vi "Hardware_CommandSTR_gen.vi"(0 "Hardware Settings":T1={"Number Samples"=5000, "Time Between Points"=0.0, "Unit"="", "Gain2 (dB)"=20, "CuttOff Freq1[MHz]"=9, "CuttOff Freq2[MHz]"=1, "Frequency"=8000000.0, "Phase"=180, "Power Level"=512, "Send Pulse"=FALSE, "Reset DDS"=FALSE, "TX CTRL"=FALSE, "RX CTRL"=FALSE, "Gain1 (dB)"=15, "Set DDS"=FALSE, "Start AQS"=FALSE} {"Gain1 (dB)" min=-5 max=45 step=1; "Power Level" max=1023 step=1; "Phase" max=270 step=90; "Frequency" min=1.0 format="%^#_6e"; "CuttOff Freq2[MHz]" min=1 max=30 step=1; "CuttOff Freq1[MHz]" min=1 max=30 step=1; "Gain2 (dB)" min=-5 max=45 step=1; "Time Between Points" min=0.0 step=1.0; "Number Samples" step=1}) -> (4 "CMD STR Array":string[](array[string]))   [LabVIEW 2011]
uses:
  Controls/Hardware Control.ctl
panel:
  in  "Send All Button":bool
  in  "On/Off 2":bool
  in  "Switch Button RX":bool
  in  "On/Off":bool
  in  "Switch Button":bool
  out "Waveform Graph":i32[][](graph)
  out "XY Graph":cluster{"magnitude":dbl[], dbl[]}(graph)
  out "XY Graph 2":cluster{"magnitude":dbl[], dbl[]}(graph)
  in  "Send Botton ADC":bool
  in  "Number Samples":u16=5000 step=1
  in  "Time Between Points":dbl min=0.0 step=1.0
  in  "ms/us Time Points":bool
  out "Real Time":ext=0.73746299999999999998
  in  "Gain (dB) 2":i8=15 min=-5 max=45 step=1
  in  "Gain (dB)":i8=20 min=-5 max=45 step=1
  in  "Numeric 2":fxp<+,12,12>
  in  "Numeric":fxp<+,12,12>
  in  "Send DAC B":bool
  in  "Send DAC A":bool
  in  "CuttOff Freq [MHz]":u8=9 min=1 max=30 step=1
  in  "CuttOff Freq[MHz]":u8=1 min=1 max=30 step=1
  in  "Send PFVGA 2":bool
  in  "Send PFVGA 1":bool
  in  "Send Pulse Botton":bool
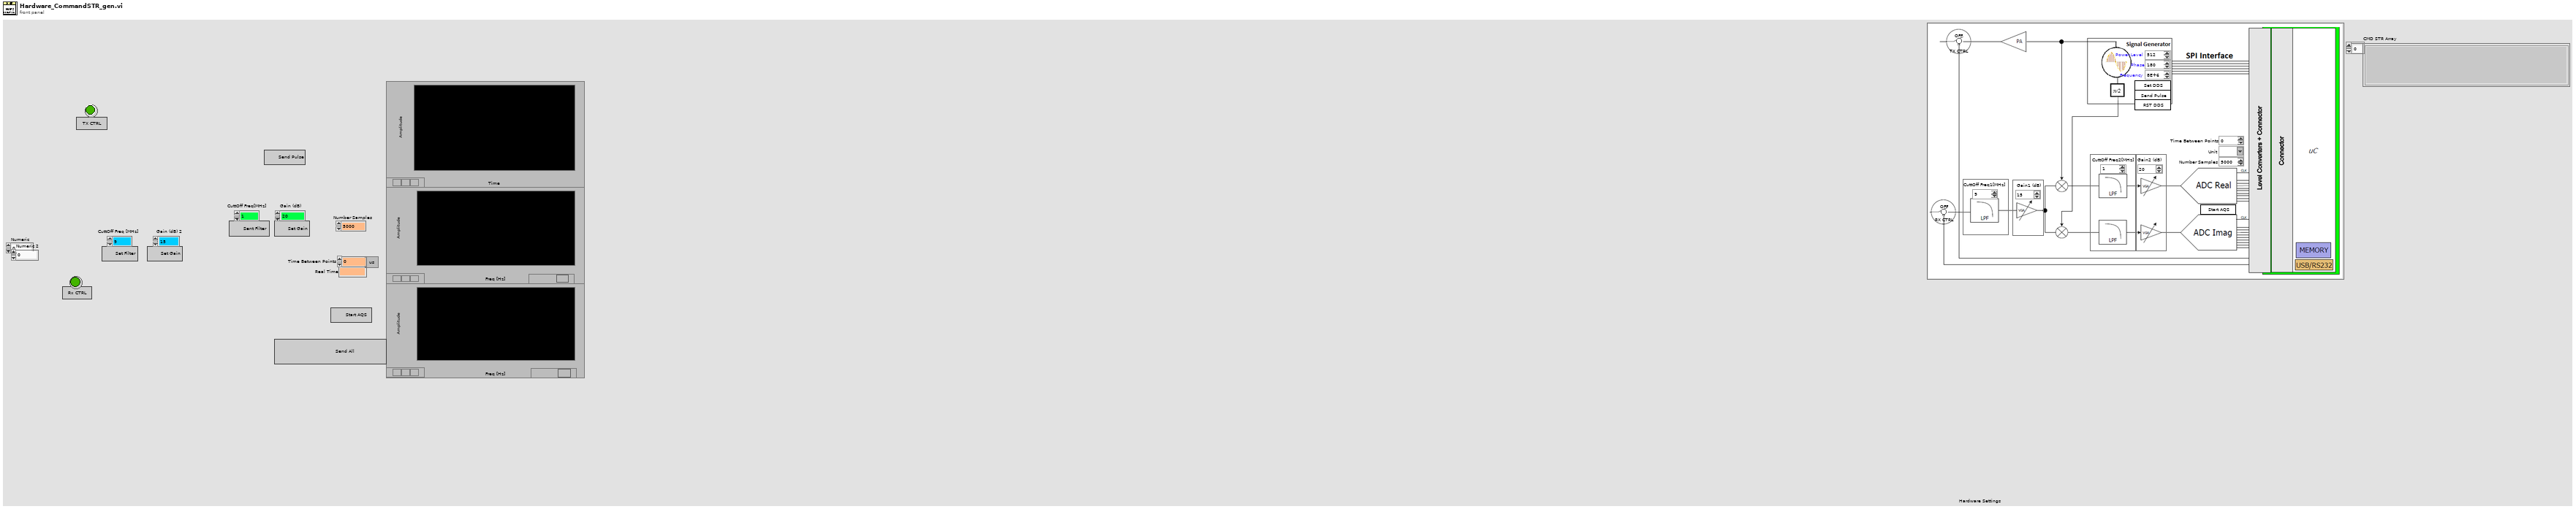
[diagram p1: front panel]
types:
  T1 = typedef "Hardware Control.ctl" = cluster{"Number Samples":u16, "Time Between Points":dbl, "Unit":string, "Gain2 (dB)":i8, "CuttOff Freq1[MHz]":u8, "CuttOff Freq2[MHz]":u8, "Frequency":dbl, "Phase":u16, "Power Level":u16, "Send Pulse":bool, "Reset DDS":bool, "TX CTRL":bool, "RX CTRL":bool, "Gain1 (dB)":i8, "Set DDS":bool, "Start AQS":bool}
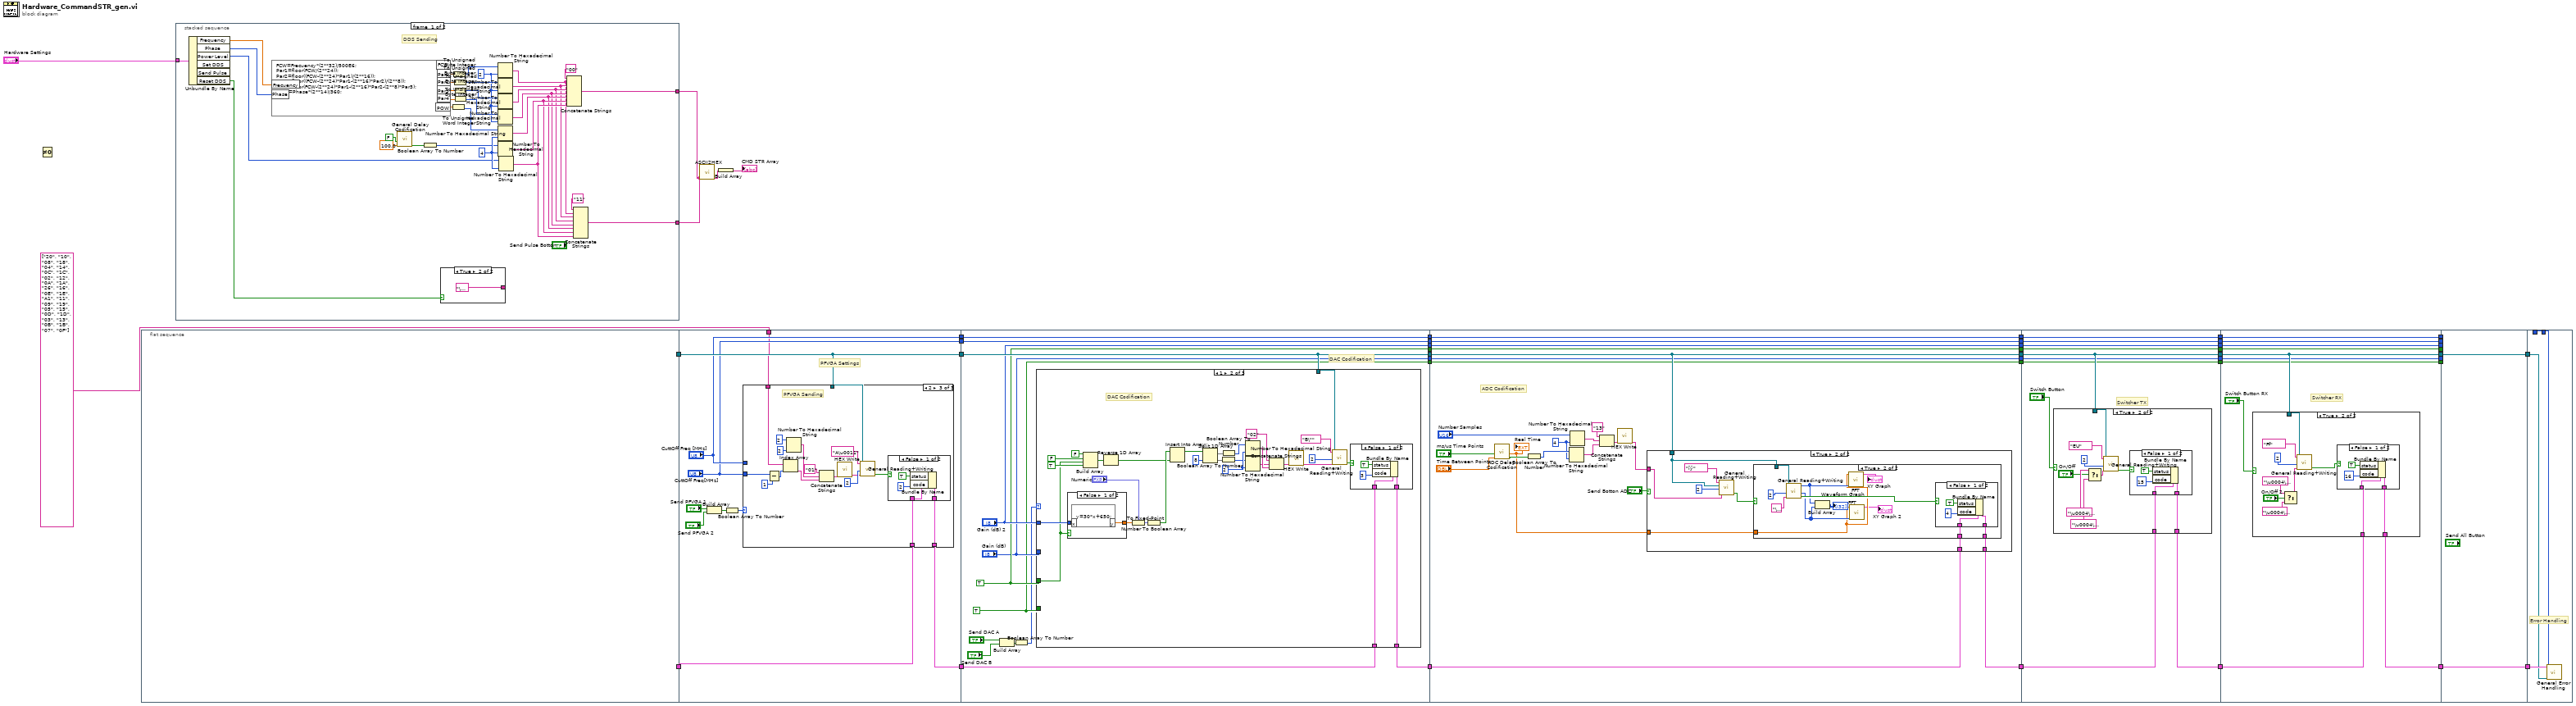
[diagram p0: block diagram]
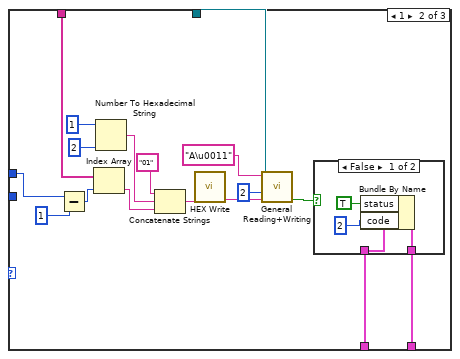
[diagram p5: hidden frame]
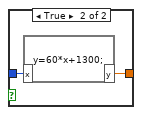
[diagram p10: hidden frame]
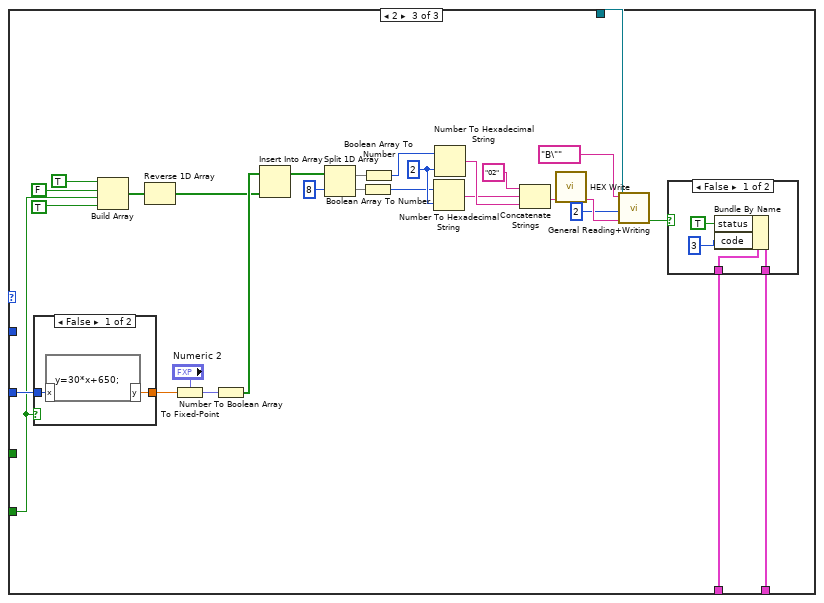
[diagram p11: hidden frame]
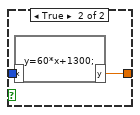
[diagram p13: hidden frame]
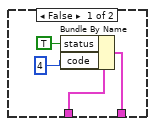
[diagram p15: hidden frame]
diagram:
  n1 = Not Equal To 0?() -> ()  [unwired: 1 in, 1 out]
  n2 = flat-sequence {
    tunnel: [_] -> w42
    tunnel: [_] -> w43
    tunnel: [w55] -> w38
    tunnel: [w54] -> w39
    tunnel: ["CuttOff Freq [MHz]"] -> w40
    tunnel: ["CuttOff Freq[MHz]"] -> w41
    tunnel: string[] ["20", "10", "08", "18", "04", "14", "0C", "1C", "02", "12", "0A", "1A", "26", "16", "0E", "1E", "A1", "11", "09", "19", "05", "15", "0D", "1D", "03", "13", "0B", "1B", "07", "0F"] ("Array") -> [w50]
    tunnel: w43 -> [w51]
    tunnel: w42 -> [w55]
    tunnel: [w113] -> w37
    tunnel: [w112] -> w36
    tunnel: [w111] -> w35
    tunnel: [w110] -> w34
    tunnel: ["Gain (dB) 2"] -> w33
    tunnel: [w108] -> w32
    tunnel: ["Gain (dB)"] -> w31
    tunnel: [w106] -> w30
    tunnel: w41 -> [w110]
    tunnel: w40 -> [w111]
    tunnel: w39 -> [w105]
    tunnel: w38 -> [w113]
    tunnel: w37 -> [w202]
    tunnel: w36 -> [w195]
    tunnel: [w205] -> w29
    tunnel: [w202] -> w28
    tunnel: w35 -> [w201]
    tunnel: [w201] -> w27
    tunnel: w34 -> [w200]
    tunnel: [w200] -> w26
    tunnel: w33 -> [w199]
    tunnel: w32 -> [w198]
    tunnel: w31 -> [w197]
    tunnel: w30 -> [w196]
    tunnel: [w199] -> w25
    tunnel: [w198] -> w24
    tunnel: [w197] -> w23
    tunnel: [w196] -> w22
    tunnel: w29 -> [w251]
    tunnel: [w250] -> w21
    tunnel: w28 -> [w249]
    tunnel: [w249] -> w20
    tunnel: w27 -> [w248]
    tunnel: w26 -> [w247]
    tunnel: [w248] -> w19
    tunnel: [w247] -> w18
    tunnel: w25 -> [w246]
    tunnel: w24 -> [w245]
    tunnel: w23 -> [w244]
    tunnel: w22 -> [w243]
    tunnel: [w246] -> w17
    tunnel: [w245] -> w16
    tunnel: [w244] -> w15
    tunnel: [w243] -> w14
    tunnel: w21 -> [w277]
    tunnel: [w276] -> w13
    tunnel: w20 -> [w275]
    tunnel: [w275] -> w12
    tunnel: w19 -> [w274]
    tunnel: w18 -> [w273]
    tunnel: [w274] -> w11
    tunnel: [w273] -> w10
    tunnel: w17 -> [w272]
    tunnel: w16 -> [w271]
    tunnel: w15 -> [w270]
    tunnel: w14 -> [w269]
    tunnel: [w272] -> w9
    tunnel: [w271] -> w8
    tunnel: [w270] -> w7
    tunnel: [w269] -> w6
    tunnel: w13 -> [w303]
    tunnel: [w303] -> w5
    tunnel: w12 -> [w295]
    tunnel: w11 -> [w302]
    tunnel: w10 -> [w301]
    tunnel: w9 -> [w300]
    tunnel: w8 -> [w299]
    tunnel: w7 -> [w298]
    tunnel: w6 -> [w297]
    tunnel: [w295] -> w4
    tunnel: w5 -> [w307]
    tunnel: w4 -> [w306]
    tunnel: _ -> [w305]
    tunnel: _ -> [w304]
    frame #0 {
    }
    frame #1 {
      # "PFVGA Settings"
      n3 = Build Array("Send PFVGA 1", "Send PFVGA 2") -> (w47:bool[])
      n4 = Boolean Array To Number(Boolean array=w47) -> (number=w46:u32)
      n5 = case shown="2" w46 {
        tunnel: w55 -> [_ w71 w92]
        tunnel: w51 -> [w56 w70 w91]
        tunnel: [w56 w69 w90] -> w54
        tunnel: "CuttOff Freq [MHz]" -> [_ w59 _]
        tunnel: w50 -> [_ w58 w82]
        tunnel: "CuttOff Freq[MHz]" -> [_ _ w81]
        frame 0, Default {
        }
        frame 1 {
          n6 = Subtract(x=w59, y=u8 1) -> (x-y=w65:u8)
          n7 = Index Array(array=w58, index=w65) -> (element=w64:string)
          n8 = Number To Hexadecimal String(1:i16 2 ("width (-)"), 2:1 ("number")) -> (0:w73:string)
          n9 = Concatenate Strings("01" ("string"), w73, w64) -> (w68:string)
          n10 = call "HEX Write.vi"("String (Normal Display)"=w68) -> ("Result string (Hex Display)"=w67:string)  [unwired: 10 in]
          n11 = call "General Reading+Writing.vi"("Write String"=w67, "Bytes to Read"=u32 2 ("Number bytes Read"), "VISA resource name"=w71, "String Seached"="A\u0011" ("search char")) -> ("Coincidence Of Character"=w60:bool)  [unwired: 4 in, 3 out]
          n12 = case shown="False" w60 {
            tunnel: w70 -> [w75 w78]
            tunnel: [w74 w78] -> w69
            frame False {
              n13 = Bundle By Name(cluster=w75, "status"=TRUE, "code"=2) -> (w74:cluster{})
            }
            frame True {
            }
          }
        }
        frame 2 {
          # "PFVGA Sending"
          n14 = Subtract(x=w81, y=u8 1) -> (x-y=w88:u8)
          n15 = Index Array(array=w82, index=w88) -> (element=w87:string)
          n16 = Number To Hexadecimal String(1:i16 2 ("width (-)"), 2:2 ("number")) -> (0:w95:string)
          n17 = Concatenate Strings("01" ("string"), w95, w87) -> (w80:string)
          n18 = call "HEX Write.vi"("String (Normal Display)"=w80) -> ("Result string (Hex Display)"=w79:string)  [unwired: 10 in]
          n19 = call "General Reading+Writing.vi"("Write String"=w79, "Bytes to Read"=u32 2 ("Number bytes Read"), "VISA resource name"=w92, "String Seached"="A\u0011" ("search char")) -> ("Coincidence Of Character"=w83:bool)  [unwired: 4 in, 3 out]
          n20 = case shown="False" w83 {
            tunnel: w91 -> [w97 w100]
            tunnel: [w96 w100] -> w90
            frame False {
              n21 = Bundle By Name(cluster=w97, "status"=TRUE, "code"=2) -> (w96:cluster{})
            }
            frame True {
            }
          }
        }
      }
    }
    frame #2 {
      w106 = TRUE ("Output Gain B")
      w108 = TRUE ("Output Gain A")
      # "DAC Codification"
      n22 = Build Array("Send DAC A", "Send DAC B") -> (w104:bool[])
      n23 = Boolean Array To Number(Boolean array=w104) -> (number=w103:u32)
      n24 = case shown="1" w103 {
        tunnel: w113 -> [_ w143 w181]
        tunnel: w105 -> [w114 w142 w180]
        tunnel: [w114 w141 w179] -> w112
        tunnel: w108 -> [_ w115 _]
        tunnel: "Gain (dB)" -> [_ _ w154]
        tunnel: "Gain (dB) 2" -> [_ w116 _]
        tunnel: w106 -> [_ _ w153]
        frame Default {
        }
        frame 1 {
          w140 = i16 2 ("width (-)")
          # "DAC Codification"
          n25 = case shown="False" w115 {
            tunnel: w116 -> [w150 w152]
            tunnel: [w149 w151] -> w129
            frame False {
              n26 = formula code="y=30*x+650;"("x"=w150) -> ("y"=w149:dbl)
            }
            frame True {
              n27 = formula code="y=60*x+1300;"("x"=w152) -> ("y"=w151:dbl)
            }
          }
          n28 = Build Array(FALSE ("element"), FALSE ("A/B"), w115, TRUE ("element")) -> (w128:bool[])
          n29 = Reverse 1D Array(array=w128) -> (reversed array=w126:bool[])
          n30 = To Fixed-Point(fixed-point type="Numeric", number=w129) -> (fixed-point=w132:fxp<+,12,12>)
          n31 = Number To Boolean Array(number=w132) -> (Boolean array=w127:bool[])
          n32 = Insert Into Array(array=w127, new element=w126) -> (w136:bool[])  [unwired: 1 in]
          n33 = Split 1D Array(array=w136, index=8) -> (first subarray=w134:bool[], second subarray=w135:bool[])
          n34 = Boolean Array To Number(Boolean array=w135) -> (number=w138:u32)
          n35 = Boolean Array To Number(Boolean array=w134) -> (number=w139:u32)
          n36 = Number To Hexadecimal String(1:w140, 2:w139) -> (0:w125:string)
          n37 = Number To Hexadecimal String(1:w140, 2:w138) -> (0:w124:string)
          n38 = Concatenate Strings("02" ("string"), w124, w125) -> (w123:string)
          n39 = call "HEX Write.vi"("String (Normal Display)"=w123) -> ("Result string (Hex Display)"=w122:string)  [unwired: 10 in]
          n40 = call "General Reading+Writing.vi"("Write String"=w122, "Bytes to Read"=u32 2 ("Number bytes Read"), "VISA resource name"=w143, "String Seached"="B\"" ("search char")) -> ("Coincidence Of Character"=w118:bool)  [unwired: 4 in, 3 out]
          n41 = case shown="False" w118 {
            tunnel: w142 -> [w145 w148]
            tunnel: [w144 w148] -> w141
            frame False {
              n42 = Bundle By Name(cluster=w145, "status"=TRUE, "code"=3) -> (w144:cluster{})
            }
            frame True {
            }
          }
        }
        frame 2 {
          w178 = i16 2 ("width (-)")
          n43 = case shown="False" w153 {
            tunnel: w154 -> [w188 w190]
            tunnel: [w187 w189] -> w167
            frame False {
              n44 = formula code="y=30*x+650;"("x"=w188) -> ("y"=w187:dbl)
            }
            frame True {
              n45 = formula code="y=60*x+1300;"("x"=w190) -> ("y"=w189:dbl)
            }
          }
          n46 = Build Array(TRUE ("element"), FALSE ("A/B"), w153, TRUE ("element")) -> (w166:bool[])
          n47 = Reverse 1D Array(array=w166) -> (reversed array=w164:bool[])
          n48 = To Fixed-Point(fixed-point type="Numeric 2", number=w167) -> (fixed-point=w170:fxp<+,12,12>)
          n49 = Number To Boolean Array(number=w170) -> (Boolean array=w165:bool[])
          n50 = Insert Into Array(array=w165, new element=w164) -> (w174:bool[])  [unwired: 1 in]
          n51 = Split 1D Array(array=w174, index=8) -> (first subarray=w172:bool[], second subarray=w173:bool[])
          n52 = Boolean Array To Number(Boolean array=w173) -> (number=w176:u32)
          n53 = Boolean Array To Number(Boolean array=w172) -> (number=w177:u32)
          n54 = Number To Hexadecimal String(1:w178, 2:w176) -> (0:w162:string)
          n55 = Number To Hexadecimal String(1:w178, 2:w177) -> (0:w163:string)
          n56 = Concatenate Strings("02" ("string"), w162, w163) -> (w161:string)
          n57 = call "HEX Write.vi"("String (Normal Display)"=w161) -> ("Result string (Hex Display)"=w160:string)  [unwired: 10 in]
          n58 = call "General Reading+Writing.vi"("Write String"=w160, "Bytes to Read"=u32 2 ("Number bytes Read"), "VISA resource name"=w181, "String Seached"="B\"" ("search char")) -> ("Coincidence Of Character"=w156:bool)  [unwired: 4 in, 3 out]
          n59 = case shown="False" w156 {
            tunnel: w180 -> [w183 w186]
            tunnel: [w182 w186] -> w179
            frame False {
              n60 = Bundle By Name(cluster=w183, "status"=TRUE, "code"=3) -> (w182:cluster{})
            }
            frame True {
            }
          }
        }
      }
    }
    frame #3 {
      w209 = i16 4 ("width (-)")
      # "ADC Codification"
      n61 = call "ADC Delay Codification.vi"("Delay"="Time Between Points", "ms/us Delay"="ms/us Time Points") -> ("Final array"=w194:bool[], "Real Time"=w191:ext)  [unwired: 8 in]
      "Real Time" <- w191
      n62 = Boolean Array To Number(Boolean array=w194) -> (number=w212:u32)
      n63 = Number To Hexadecimal String(1:w209, 2:w212) -> (0:w211:string)
      n64 = Number To Hexadecimal String(1:w209, 2:"Number Samples") -> (0:w210:string)
      n65 = Concatenate Strings("13" ("string"), w210, w211) -> (w204:string)
      n66 = call "HEX Write.vi"("String (Normal Display)"=w204) -> ("Result string (Hex Display)"=w203:string)  [unwired: 10 in]
      n67 = case shown="True" "Send Botton ADC" {
        tunnel: w203 -> [_ w218]
        tunnel: w202 -> [_ w215]
        tunnel: [w213 w221] -> w205
        tunnel: w195 -> [w213 w216]
        tunnel: w191 -> [_ w214]
        frame False {
        }
        frame True {
          n68 = call "General Reading+Writing.vi"("Write String"=w218, "Bytes to Read"=u32 2 ("Number bytes Read"), "VISA resource name"=w215, "String Seached"="ïÿ" ("search char")) -> ("Coincidence Of Character"=w217:bool)  [unwired: 4 in, 3 out]
          n69 = case shown="True" w217 {
            tunnel: w215 -> [_ w236]
            tunnel: w216 -> [w223 w234]
            tunnel: [w222 w233] -> w221
            tunnel: w214 -> [_ w228]
            frame False {
              n70 = Bundle By Name(cluster=w223, "status"=TRUE, "code"=4) -> (w222:cluster{})
            }
            frame True {
              n71 = call "General Reading+Writing.vi"("Write String"="\u0014", "Bytes to Read"=u32 2 ("Number Of Bytes to Read"), "VISA resource name"=w236) -> ("Coincidence Of Character"=w235:bool, "Imag Data"=w230:i32[], "Real Data"=w231:i32[])  [unwired: 5 in, 1 out]
              n72 = Build Array(w231, w230) -> (→"Waveform Graph":i32[][])
              n73 = call "FFT.vi"("Input Array"=w231, "Delay Sample"=w228) -> ("FFT Graph"=→"XY Graph":cluster{"magnitude":dbl[], dbl[]})  [unwired: 8 in, 1 out]
              n74 = call "FFT.vi"("Input Array"=w230, "Delay Sample"=w228) -> ("FFT Graph"=→"XY Graph 2":cluster{"magnitude":dbl[], dbl[]})  [unwired: 8 in, 1 out]
              n75 = case shown="False" w235 {
                tunnel: w234 -> [w239 w242]
                tunnel: [w238 w242] -> w233
                frame False {
                  n76 = Bundle By Name(cluster=w239, "status"=TRUE, "code"=4) -> (w238:cluster{})
                }
                frame True {
                }
              }
            }
          }
        }
      }
    }
    frame #4 {
      # "Switcher TX"
      n77 = case shown="True" "Switch Button" {
        tunnel: w249 -> [_ w260]
        tunnel: w251 -> [w253 w259]
        tunnel: [w253 w258] -> w250
        frame False {
        }
        frame True {
          n78 = Select(t="\u0004\u0000\u0000", s="On/Off", f="\u0004\u0000\u0001") -> (s? t:f=w255:string)
          n79 = call "General Reading+Writing.vi"("Write String"=w255, "Bytes to Read"=u32 2 ("Number bytes Read"), "VISA resource name"=w260, "String Seached"="EU" ("search char")) -> ("Coincidence Of Character"=w261:bool)  [unwired: 4 in, 3 out]
          n80 = case shown="False" w261 {
            tunnel: w259 -> [w265 w268]
            tunnel: [w264 w268] -> w258
            frame False {
              n81 = Bundle By Name(cluster=w265, "status"=TRUE, "code"=15) -> (w264:cluster{})
            }
            frame True {
            }
          }
        }
      }
    }
    frame #5 {
      # "Switcher RX"
      n82 = case shown="True" "Switch Button RX" {
        tunnel: w275 -> [_ w284]
        tunnel: w277 -> [w279 w286]
        tunnel: [w279 w285] -> w276
        frame False {
        }
        frame True {
          n83 = Select(t="\u0004\u0001\u0000", s="On/Off 2", f="\u0004\u0001\u0001") -> (s? t:f=w281:string)
          n84 = call "General Reading+Writing.vi"("Write String"=w281, "Bytes to Read"=u32 2 ("Number bytes Read"), "VISA resource name"=w284, "String Seached"="Ff" ("search char")) -> ("Coincidence Of Character"=w287:bool)  [unwired: 4 in, 3 out]
          n85 = case shown="False" w287 {
            tunnel: w286 -> [w291 w294]
            tunnel: [w290 w294] -> w285
            frame False {
              n86 = Bundle By Name(cluster=w291, "status"=TRUE, "code"=16) -> (w290:cluster{})
            }
            frame True {
            }
          }
        }
      }
    }
    frame #6 {
    }
    frame #7 {
      # "Error Handling"
      n87 = call "General Error Handling.vi"("VISA resource name"=w306, "timeout (10sec)"=w304, "baud rate (9600)"=w305, "error IO"=w307) -> ()  [unwired: 8 in]
    }
  }
  n88 = stacked-sequence {
    tunnel: "Hardware Settings" -> [w339 _]
    tunnel: w1 -> [w316 _]
    tunnel: [w315 _] -> w1
    frame #0 {
      w338 = i16 4 ("width (-)")
      w325 = i16 2 ("width (-)")
      # "DDS Sending"
      n89 = Unbundle By Name(w339) -> ("Frequency"=w314:dbl, "Phase"=w313:u16, "Power Level"=w312:u16, "Reset DDS"=w308:bool)  [unwired: 2 out]
      n90 = formula code="FCW=Frecuency*(2**32)/500E6;\nPar1=floor(FCW/(2**24));\nPar2=floor((FCW-(2**24)*Par1)/(2**16));\nPar3=floor((FCW-(2**24)*Par1-(2**16)*Par2)/(2**8));\nPar4=floor(FCW-(2**24)*Par1-(2**16)*Par2-(2**8)*Par3);\nPOW=Phase*(2**14)/360;"("Frecuency"=w314, "Phase"=w313) -> ("Par1"=w323:dbl, "Par2"=w322:dbl, "Par3"=w321:dbl, "Par4"=w320:dbl, "POW"=w318:dbl)  [unwired: 1 out]
      n91 = call "General Delay Codification.vi"("Delay"=100.0, "ms/us Delay"=FALSE) -> ("Final array"=w311:bool[])  [unwired: 8 in, 1 out]
      n92 = Boolean Array To Number(Boolean array=w311) -> (number=w317:u32)
      n93 = case shown="True" w308 {
        tunnel: [_ "\u0015" ("Result string (Hex Display)")] -> _
        frame False {
        }
        frame True {
        }
      }
      n94 = To Unsigned Word Integer(number=w318) -> (unsigned 16bit integer=w319:u16)
      n95 = To Unsigned Byte Integer(number=w323) -> (unsigned 8bit integer=w329:u8)
      n96 = To Unsigned Byte Integer(number=w322) -> (unsigned 8bit integer=w328:u8)
      n97 = To Unsigned Byte Integer(number=w321) -> (unsigned 8bit integer=w327:u8)
      n98 = To Unsigned Byte Integer(number=w320) -> (unsigned 8bit integer=w326:u8)
      n99 = Number To Hexadecimal String(1:w325, 2:w329) -> (0:w330:string)
      n100 = Number To Hexadecimal String(1:w325, 2:w328) -> (0:w331:string)
      n101 = Number To Hexadecimal String(1:w325, 2:w327) -> (0:w332:string)
      n102 = Number To Hexadecimal String(1:w325, 2:w326) -> (0:w333:string)
      n103 = Number To Hexadecimal String(1:w338, 2:w319) -> (0:w334:string)
      n104 = Number To Hexadecimal String(1:w338, 2:w317) -> (0:w335:string)
      n105 = Number To Hexadecimal String(1:w338, 2:w312) -> (0:w336:string)
      n106 = Concatenate Strings("00" ("string"), w330, w331, w332, w333, w334, w335, w336) -> (w316:string)
      n107 = Concatenate Strings("11" ("string"), w330, w331, w332, w333, w334, w335, w336) -> (w315:string)
    }
    frame #1 {
    }
  }
  n108 = call "ASCII2HEX.vi"("String (Normal Display)"=w1) -> ("Result string (Hex Display)"=w45:string)  [unwired: 10 in]
  n109 = Build Array(w45) -> (→"CMD STR Array":string[])
